vi "NISE.remote.Commit NVMEM (Core).vi"(7 "nvmem type":T1, 8 "error in (no error)":errorcluster, 10 "resources":string, 11 "SLSC Remote in":refnum<class "SLSC Interface.lvclass">) -> (0 "error out":errorcluster, 3 "SLSC Remote out":refnum<class "SLSC Interface.lvclass">)   [LabVIEW 2016, in "SLSC Interface.lvclass"]
uses:
  SLSC Interface Class/SLSC Interface.lvclass
  SLSC Interface Class/NISE.nvmem type.ctl
  SLSC Interface Class/SLSC Interface.lvclass/SLSC Interface.ctl
  SLSC Interface Class/NISE.Read client handle.vi
  SLSC Interface Class/NISE.Read URL.vi
  SLSC Interface Class/NISE.Read session.vi
  <vilib>/httpClient/POSTBuffer.vi
  <vilib>/httpClient/LabVIEWHTTPClient.lvlib
  <vilib>/NI/JSON Support for LabVIEW/JSON Value/JSON Value.lvclass
  <vilib>/NI/NI JSONRPC Server Framework/Classes/Client/JSONRPC Client.lvclass
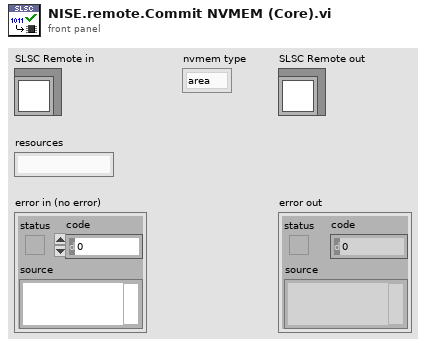
[diagram p1: front panel]
types:
  T1 = typedef "SLSC Interface.lvclass/NISE.nvmem type.ctl" = enum16{"area", "device", "session"}
  T2 = typedef "LabVIEWHTTPClient.lvlib/ClientHandle.ctl" = refnum<k1>
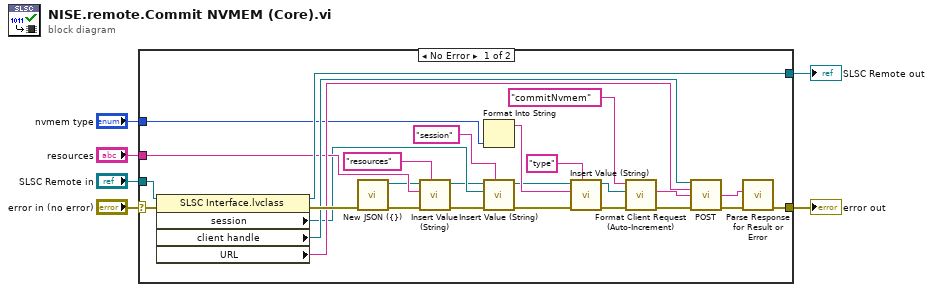
[diagram p0: block diagram]
diagram:
  n1 = case shown="No Error" "error in (no error)" {
    selector: "error in (no error)" -> [w31 w34]
    tunnel: "resources" -> [w15 _]
    tunnel: "SLSC Remote in" -> [w33 w35]
    tunnel: [w32 w35] -> w4
    tunnel: [w20 w34] -> w2
    tunnel: "nvmem type" -> [w16 _]
    frame No Error {
      n2 = property class="SLSC Interface.lvclass"(reference=w33, error in=w31) -> (reference out=w32:refnum<class "SLSC Interface.lvclass">, error out=w30:errorcluster, "session"=w14:refnum<k21>, "client handle"=w25:T2, "URL"=w24:string)
      n3 = call <vilib>:"New JSON ({}).vi"("error in (no error)"=w30) -> ("error out"=w29:errorcluster, "JSON Value out"=w9:refnum<class "JSON Value.lvclass">)  [unwired: 9 in]
      n4 = call <vilib>:"Insert Value (String).vi"("key"="resources" ("Name"), "error in (no error)"=w29, "value"=w15, "JSON Value in"=w9) -> ("error out"=w28:errorcluster, "JSON Value out"=w8:refnum<class "JSON Value.lvclass">)  [unwired: 5 in, 1 out]
      n5 = Format Into String(w16) -> (resulting string=w13:string)  [unwired: 3 in, 1 out]
      n6 = call <vilib>:"Insert Value (String).vi"("key"="session" ("Name"), "error in (no error)"=w28, "value"=w14, "JSON Value in"=w8) -> ("error out"=w18:errorcluster, "JSON Value out"=w7:refnum<class "JSON Value.lvclass">)  [unwired: 5 in, 1 out]
      n7 = call <vilib>:"Insert Value (String).vi"("key"="type" ("Name"), "error in (no error)"=w18, "value"=w13, "JSON Value in"=w7) -> ("error out"=w17:errorcluster, "JSON Value out"=w19:refnum<class "JSON Value.lvclass">)  [unwired: 5 in, 1 out]
      n8 = call <vilib>:"Format Client Request (Auto-Increment).vi"("error in (no error)"=w17, "JSON Value in"=w19, "method"="commitNvmem") -> ("error out"=w23:errorcluster, "Request String"=w26:string)  [unwired: 7 in]
      n9 = call-poly <vilib>:"POST.vi"("client handle"=w25, "url"=w24, "buffer"=w26, "error in (no error)"=w23) -> ("body"=w22:string, "error out"=w21:errorcluster)  [unwired: 8 in, 2 out]
      n10 = call <vilib>:"Parse Response for Result or Error.vi"("error in"=w21, "Response String In"=w22) -> ("error out"=w20:errorcluster)  [unwired: 7 in, 2 out]
    }
    frame Error {
    }
  }
  "error out" <- w2
  "SLSC Remote out" <- w4
